vi "UIWriteCtrlIndex.vi"(8 "error in":errorcluster, 9 "Control Value":variant, 10 "Index":i32, 11 "UI Ref cluster in":T1) -> (0 "error out":errorcluster, 3 "UI Ref cluster out":T1)   [LabVIEW 2025, in "UI_Library.lvlib" / "UI_Library.lvclass"]
doc: "Write new value to a Control by index if found"
uses:
  UI_Library.lvclass
  Controls/UI_RefCluster.ctl
  <vilib>/Utility/Data Type/Type Definitions/Data Type.ctl
  UI_Library.lvlib
  <vilib>/Utility/Data Type/NI_Data Type.lvlib
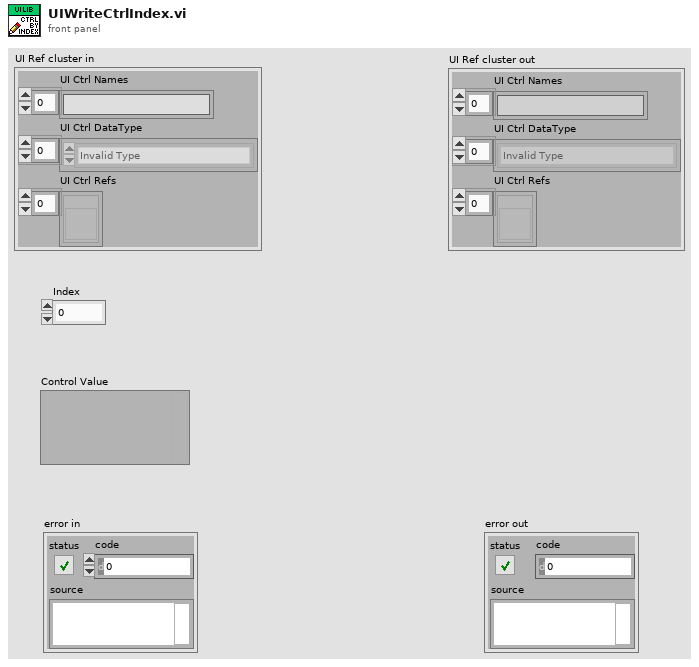
[diagram p1: front panel]
types:
  T1 = typedef "UI_Library.lvlib/UI_RefCluster.ctl" = cluster{"UI Ctrl Names":string[], "UI Ctrl DataType":T2[], "UI Ctrl Refs":refnum<vi>[]}
  T2 = typedef "NI_Data Type.lvlib/Data Type.ctl" = enum8{"Invalid Type", "Void", "I8", "I16", "I32", "I64", "U8", "U16", "U32", "U64", "Single Float", "Double Float", "Extended Float", "Single Complex", "Double Complex", "Extended Complex", "Enum U8", "Enum U16", "Enum U32", "Enum U64", "Single Float With Unit", "Double Float With Unit", "Extended Float With Unit", "Single Complex with Unit", "Double Complex with Unit", "Extended Complex with Unit", "Boolean", "String", "Path", "Picture", "Tag", "Array", "Cluster", "Variant", "LV Variant", "Waveform", "Timestamp", "Digital Waveform", "Digital Data", "ExpressData", "Refnum", "External Data", "VI", "Poly VI", "LabVIEW Class Instance", "Fixed Point", "Set Collection", "Map Collection"}
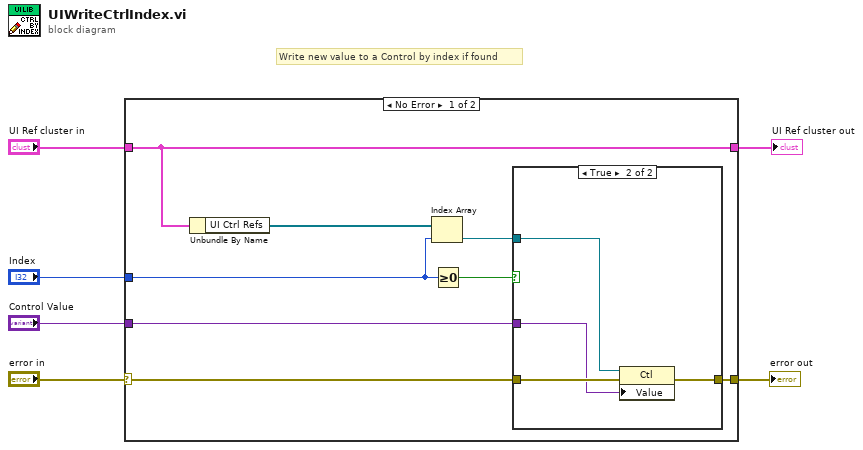
[diagram p0: block diagram]
diagram:
  # "Write new value to a Control by index if found"
  n1 = case shown="No Error" "error in" {
    selector: "error in" -> [w11 w21]
    tunnel: [w10 w21] -> w6
    tunnel: "Control Value" -> [w9 _]
    tunnel: [w8 w20] -> w3
    tunnel: "UI Ref cluster in" -> [w8 w20]
    tunnel: "Index" -> [w7 _]
    frame No Error {
      n2 = Unbundle By Name(w8) -> ("UI Ctrl Refs"=w13:refnum<vi>[])
      n3 = Index Array(array=w13, index=w7) -> (element=w12:refnum<vi>)
      n4 = Greater Or Equal To 0?(x=w7) -> (x >= 0?=w14:bool)
      n5 = case shown="True" w14 {
        tunnel: w12 -> [_ w19]
        tunnel: w11 -> [w15 w17]
        tunnel: [w15 w18] -> w10
        tunnel: w9 -> [_ w16]
        frame False {
        }
        frame True {
          n6 = property class="Ctl"(reference=w19, error in=w17, "Value"=w16) -> (error out=w18:errorcluster)  [unwired: 1 out]
        }
      }
    }
    frame Error {
    }
  }
  "error out" <- w6
  "UI Ref cluster out" <- w3
